vi "TruncDBL.vi"(5 "Decimal places":i8, 6 "Number":dbl format="%#.10f") -> (2 "Truncated number":dbl format="%#.10f")   [LabVIEW 2017, in "GPNumeric.lvlib"]
doc: "Truncates <B>Number</B> to a number of <B>Decimal places</B>.\n\nYou can set <B>Decimal places</B> to a negative number to truncate to nearest 10, nearest 100 and so on. E.g. to truncate 782.402 to the nearest hundred, you set <B>Decimal places</B> to -2 and the <B>Truncated number</B> will be 700.\n\nThis VI is inlined.\n\nSteen Schmidt\nGPower\n5/4 2014"
uses:
  GPNumeric.lvlib
panel:
  # "Copyright © 2014\nGPower\nSee enclosed license file for terms and conditions"
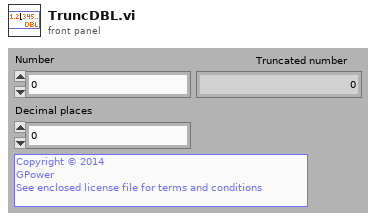
[diagram p1: front panel]
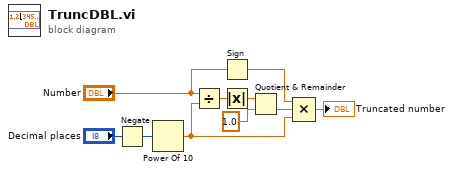
[diagram p0: block diagram]
diagram:
  n1 = Negate(x="Decimal places") -> (-x=w10:i8)
  n2 = Power Of 10(x=w10) -> (10^x=w4:dbl)
  n3 = Divide(x="Number", y=w4) -> (x/y=w9:dbl)
  n4 = Sign(1:"Number") -> (0:w2:dbl)
  n5 = Absolute Value(x=w9) -> (abs(x)=w6:dbl)
  n6 = Quotient & Remainder(x=w6, y=1.0) -> (floor(x/y)=w3:dbl)  [unwired: 1 out]
  n7 = Compound Arithmetic op=MULTIPLY(w2, w3, w4) -> (→"Truncated number":dbl)
